vi "EXA_acceptCommand_EnterControl.vi"(8 "error in (no error)":errorcluster, 11 "command_EnterControl_Ctl":T1) -> (0 "error out":errorcluster, 2 "function return":i32, 3 "command_EnterControl_Ctl out":T1)   [LabVIEW 2016, in "SALLV_EXA.lvlib"]
doc: "int EXA_shm_acceptCommand_EnterControlLV(EXA_command_EnterControlLV *command_EnterControl_Ctl );"
uses:
  SALLV_EXA.lvlib
  DataTypes/command_EnterControl.ctl
  SALLV_EXA.so
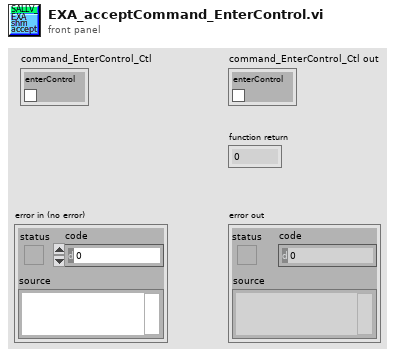
[diagram p1: front panel]
types:
  T1 = typedef "SALLV_EXA.lvlib/command_EnterControl.ctl" = cluster{"enterControl":bool}
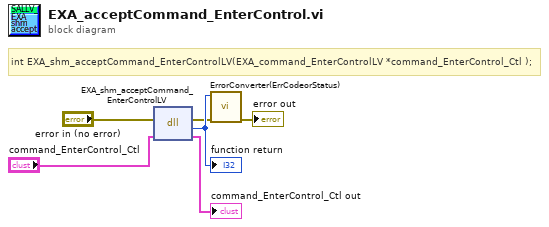
[diagram p0: block diagram]
diagram:
  # "int EXA_shm_acceptCommand_EnterControlLV(EXA_command_EnterControlLV *command_EnterControl_Ctl );"
  n1 = dll-call lib="home/andres/Desktop/SAL_EXA2/SALLV_EXA.*" fn="EXA_shm_acceptCommand_EnterControlLV"(error in="error in (no error)", "command_EnterControl_Ctl"="command_EnterControl_Ctl") -> (error out=w2:errorcluster, w6:i32, "command_EnterControl_Ctl"=→"command_EnterControl_Ctl out":T1)  [unwired: 2 in, 1 out]
  "function return" <- w6
  n2 = call "ErrorConverter(ErrCodeorStatus).vi"("error in (no error)"=w2, "error code"=w6) -> ("error out"=→"error out":errorcluster)  [unwired: 9 in]
